vi "CSM - Read Key Names.vi"(5 "Section Name (\"\" as Default)":string, 7 "error in (no error)":errorcluster) -> (1 "error out":errorcluster, 3 "Keys":string[](array[string]))   [LabVIEW 2017, in "INI-Static-Variable-Support.lvlib"]
uses:
  INI-Static-Variable-Support.lvlib
  _fgv-oper.ctl
  <userlib>/_NEVSTOP/Communicable State Machine(CSM)/_Support/ChangeFlag/ChangeFlag-Read.vi
  <userlib>/_NEVSTOP/Communicable State Machine(CSM)/_Support/ChangeFlag/ChangeFlagDB.vi
  <userlib>/_NEVSTOP/Communicable State Machine(CSM)/Communicable State Machine.lvlib
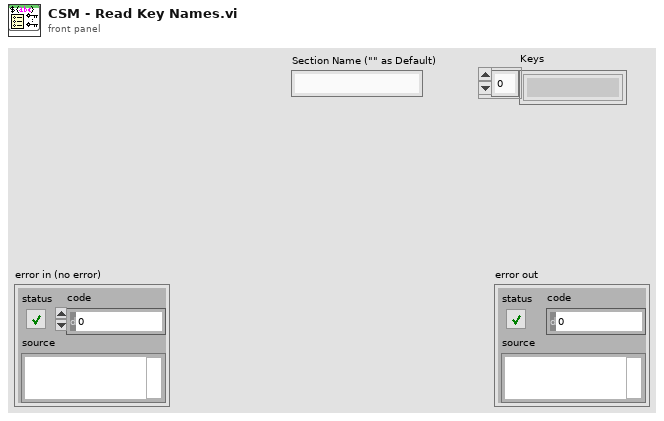
[diagram p1: front panel]
types:
  T1 = typedef "INI-Static-Variable-Support.lvlib/_fgv-oper.ctl" = enum16{"Read", "Write", "Sync", "Sessions", "List Keys", "Load", "List Files", "List Variables", "List Permanent Variables", "Mark Temp Variable as Permenent", "unload", "INIConfig(Memory)", "Reset", "Restore Variable Value"}
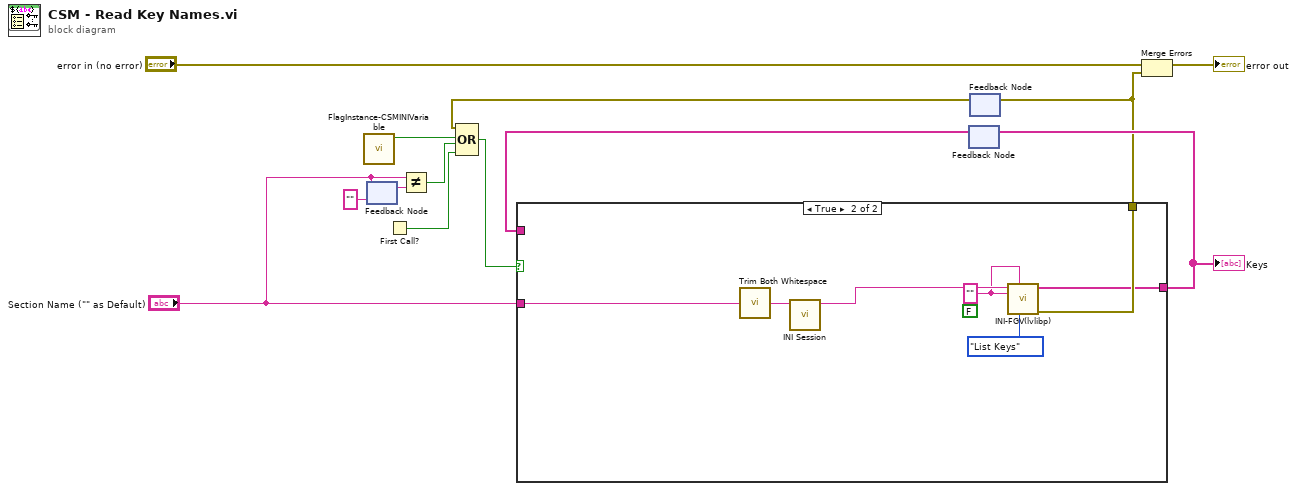
[diagram p0: block diagram]
diagram:
  n1 = call "FlagInstance-CSMINIVariable.vi"() -> ("Changed"=w1:bool)  [unwired: 10 in, 1 out]
  n2 = feedback #1("" ("Section Name(\"\" as Default)")) -> (w11:string)
  n3 = feedback-in #1("Section Name (\"\" as Default)") -> ()
  n4 = First Call?() -> (First Call?: T/F=w2:bool)
  n5 = Not Equal?(x="Section Name (\"\" as Default)", y=w11) -> (x != y?=w9:bool)
  n6 = feedback #2() -> (w7:string[])  [unwired: 1 in]
  n7 = feedback #3() -> (w5:errorcluster)  [unwired: 1 in]
  n8 = Compound Arithmetic op=OR(w5, w1, w9, w2) -> (w4:bool)
  n9 = case shown="True" w4 {
    tunnel: [_ w20] -> w6
    tunnel: [w14 w19] -> w8
    tunnel: "Section Name (\"\" as Default)" -> [_ w18]
    tunnel: w7 -> [w14 _]
    frame False {
    }
    frame True {
      w15 = "" (">> Default Value >>")
      (unwired) FALSE ("Raw String? (F)")
      n10 = call <userlib>:"Trim Both Whitespace.vi"("String"=w18) -> ("Trimmed String"=w17:string)  [unwired: 1 in]
      n11 = call "INI Session.vi"("Section Name(\"\" as Default)"=w17) -> ("App.Name"=w16:string)  [unwired: 10 in]
      n12 = call "INI-FGV(lvlibp).vi"("Enum"=_fgv-oper."List Keys", "Prefered Section"=w15, ">> Default Value >>"=w15, ">> Variable Name >>"=w16) -> ("error out"=w20:errorcluster, "Array"=w19:string[])  [unwired: 4 in, 2 out]
    }
  }
  "Keys" <- w8
  n13 = feedback-in #2(w8) -> ()
  n14 = feedback-in #3(w6) -> ()
  n15 = Merge Errors("error in (no error)", w6) -> (→"error out":errorcluster)
